vi "video.get_ingest_status.vi"(8 "error in":errorcluster, 10 "Video RID":string, 11 "Nominal Client in":refnum<class "Nominal Client.lvclass">) -> (0 "error out":errorcluster, 1 "Progress (0-1)":dbl, 2 "Status":string, 3 "Nominal Client out":refnum<class "Nominal Client.lvclass">)   [LabVIEW 2018, in "Nominal Client.lvclass"]
doc: "The returned status will be:\nsuccess, error, or inProgress"
uses:
  Nominal Client.lvclass
  3ce23808-1dd2-45d8-8215-d591b3b9a39c.vi
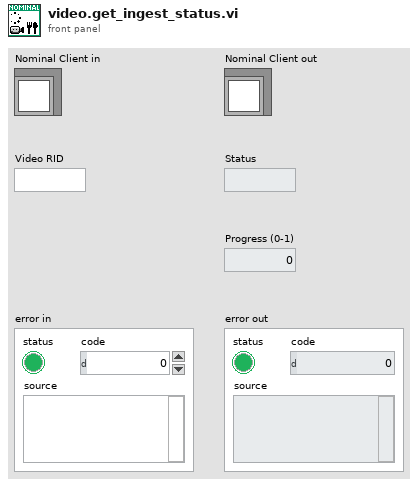
[diagram p1: front panel]
types:
  T1 = cluster{"type":string, "error":cluster{"errors":cluster{"errorType":string, "message":string}[]}, "inProgress":dbl}
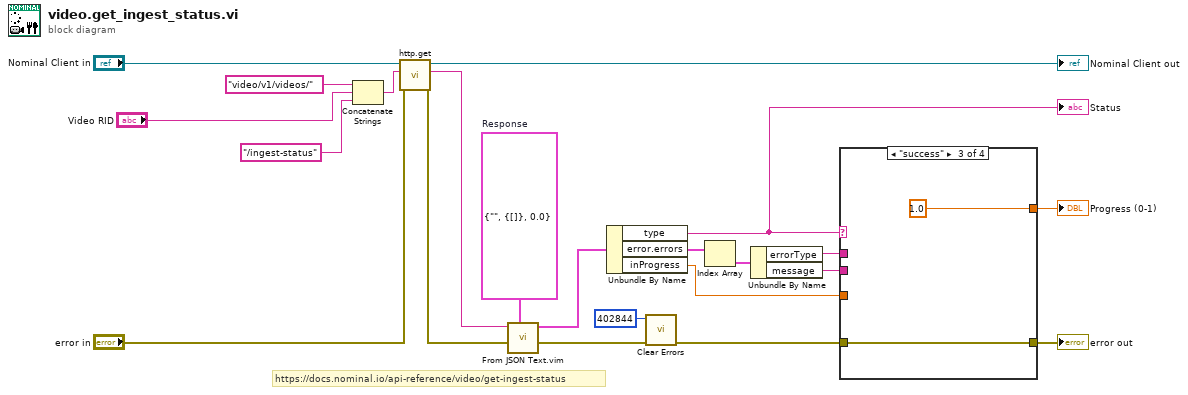
[diagram p0: block diagram]
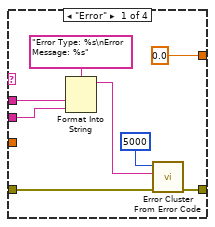
[diagram p2: hidden frame]
diagram:
  w8 = T1 {"type"="", "error"={"errors"=[]}, "inProgress"=0.0}  # Response
  # "https://docs.nominal.io/api-reference/video/get-ingest-status"
  n1 = Concatenate Strings("video/v1/videos/" ("Path"), "Video RID", "/ingest-status" ("Path")) -> (w20:string)
  n2 = call "http.get.vi"("error in"="error in", "Path"=w20, "Nominal Client in"="Nominal Client in") -> ("error out"=w15:errorcluster, "Response"=w16:string, "Nominal Client out"=→"Nominal Client out":refnum<class "Nominal Client.lvclass">)  [unwired: 5 in, 1 out]
  n3 = call "From JSON Text.vim"("Data Type and Default Value"=w8, "error in (no error)"=w15, "JSON"=w16) -> ("error out"=w18:errorcluster, "Data out"=w14:T1)  [unwired: 7 in]
  n4 = Unbundle By Name(w14) -> ("type"=w3:string, "error.errors"=w7:cluster{"errorType":string, "message":string}[], "inProgress"=w1:dbl)
  "Status" <- w3
  n5 = call <vilib>:"Clear Errors.vi"("error in (no error)"=w18, "specific error code to clear (0: all)"=402844) -> ("error out"=w17:errorcluster)  [unwired: 4 in, 1 out]
  n6 = Index Array(array=w7) -> (element=w6:cluster{"errorType":string, "message":string})  [unwired: 1 in]
  n7 = Unbundle By Name(w6) -> ("errorType"=w5:string, "message"=w4:string)
  n8 = case shown="\"success\"" w3 {
    tunnel: w17 -> [w29 w31 w33 w35]
    tunnel: [w30 w31 w33 w35] -> w9
    tunnel: w5 -> [w25 _ _ _]
    tunnel: w4 -> [w24 _ _ _]
    tunnel: [0.0 w32 1.0 _] -> w2
    tunnel: w1 -> [_ w32 _ _]
    frame "Error" {
      n9 = Format Into String(format string="Error Type: %s\nError Message: %s", w25, w24) -> (resulting string=w26:string)  [unwired: 2 in, 1 out]
      n10 = call <vilib>:"Error Cluster From Error Code.vi"("error in (no error)"=w29, "error message (\"\")"=w26, "error code (0)"=5000) -> ("error out"=w30:errorcluster)  [unwired: 6 in]
    }
    frame "inProgress" {
    }
    frame "success" {
    }
    frame Default {
    }
  }
  "error out" <- w9
  "Progress (0-1)" <- w2
